vi "GUI_Cameras_v1.2.0_TEMP.vi"() -> ()   [LabVIEW 2013]
uses:
  <vilib>/vision/NI_Vision_Development_Module.lvlib
  <vilib>/Analysis/NI_AALBase.lvlib
  <vilib>/Analysis/baseanly.llb/Mean (DBL).vi
  <vilib>/Utility/miscctls.llb/LVRectTypeDef.ctl
panel:
  out "data array":dbl[](array[numeric])
  out "Guppy Y":dbl=985.6842015448223
  out "Guppy X":dbl=985.6842015448223
  out "M3 X":dbl=985.6842015448223
  out "M3 Y":dbl=985.6842015448223
  out "Image (Guppy)":T1(plugin-control)
  out "Image (OAP)":T1(plugin-control)
  in  "ROI":T2={"Global Rectangle"=[217, 150, 349, 397], "Contours"=[{"Contour Type"=0, "ROI Type"=3, "Points"=[217, 150, 349, 397]}, {"Contour Type"=0, "ROI Type"=3, "Points"=[382, 143, 522, 397]}, {"Contour Type"=0, "ROI Type"=3, "Points"=[555, 160, 687, 390]}]}
  out "Boolean":bool=TRUE
  out "time string":string="2:08 PM"
  in  "Search Decimal Separator":bool=TRUE
  out "Output value":dbl=2.5400000000000005 format="%.2f"
  in  "LCD/LED (LCD)":bool
  out "Segments status":T3(array[cluster])=[{TRUE, TRUE, FALSE, TRUE, TRUE, FALSE, TRUE}, {TRUE, FALSE, TRUE, TRUE, FALSE, TRUE, TRUE}, {FALSE, TRUE, TRUE, FALSE, FALSE, TRUE, TRUE}]
  out "error out 2":errorcluster
  in  "Threshold":dbl=3.0 format="%.2f"
  out "Zoom changed":bool
  out "Zoom old":cluster{"X":sgl, "Y":sgl}={"X"=1.2111253, "Y"=1.773196}
  out "MaxCounts":dbl(slide)=255.0 scale=0.0..256.0
  out "ratio(h)":bool=TRUE
  out "fixsize":bool
  out "Change Ratio":cluster{"X":sgl, "Y":sgl}={"X"=0.41283923, "Y"=0.28197673}
  out "old Panel Bounds":T4={"Left"=2, "Top"=-1034, "Right"=1328, "Bottom"=-402}
  in  "shotnumber":i32=32
  in  "gain":dbl
  in  "exposure":dbl=0.032 caption="Exposure"
  in  "save":bool
  in  "trigger":bool
  in  "triggerdelay":dbl
  out "error (h)":bool
  in  "Main Tap":T5(tab)=enum."Time"
  out "Image (IMAQ)":T1(plugin-control)
  out "output cluster":cluster{dbl[], dbl[]}[](graph)
  out "local Port":u16=65401
  out "Remote Host":string="192.168.10.115"
  out "port or service name":u16=65417
  in  "timeout ms (slow resp)":i32=500
  in  "reset":bool
  out "All Devices (h)":string[](array[string])=["StagingDiodeMonitor", "StagingFocusBeam1", "StagingFocusBeam2", "StagingGuppy", "StagingM1Far", "StagingM1Near", "StagingM3Far", "StagingOAP1Far", "StagingOAP1Near", "StagingOAP2Far", "StagingOAP2Near", "TS-InputNearField", "TS-Mode1"]
  out "centroidy":dbl=447.895874
  out "fast ID (h)":refnum<k16>
  out "slow ID (h)":refnum<k16>
  out "error out":errorcluster
  out "connections (hidden)":variant[](array[variant])=[variant(refnum<k16> refnum), variant(refnum<k16> refnum)]
  in  "time to wait (main loop)":i32=10
  in  "time to wait (TCP)":i32=10
  out "Data String":string="exposure,0.032000\r\ntrigger,off\r\nsave,off\r\ngain,0.000000\r\ntriggerdelay,0.000000\r\nlocalsavingpath,c:\\temp\r\ncentroidy,447.895874\r\ncentroidy,447.895874\r\n"
  in  "send":bool
  in  "localsavingpath":path=path "c:/temp"
  out "centroidy":dbl=447.895874
  out "Image (array)":u8[][](graph)
  out "Device Name (h)":string="StagingFocusBeam1"
  out "stop":bool
  out "error message":string
  out "image connection":bool=TRUE
  out "data connection ok":bool=TRUE
  # "Data"
  # "Image"
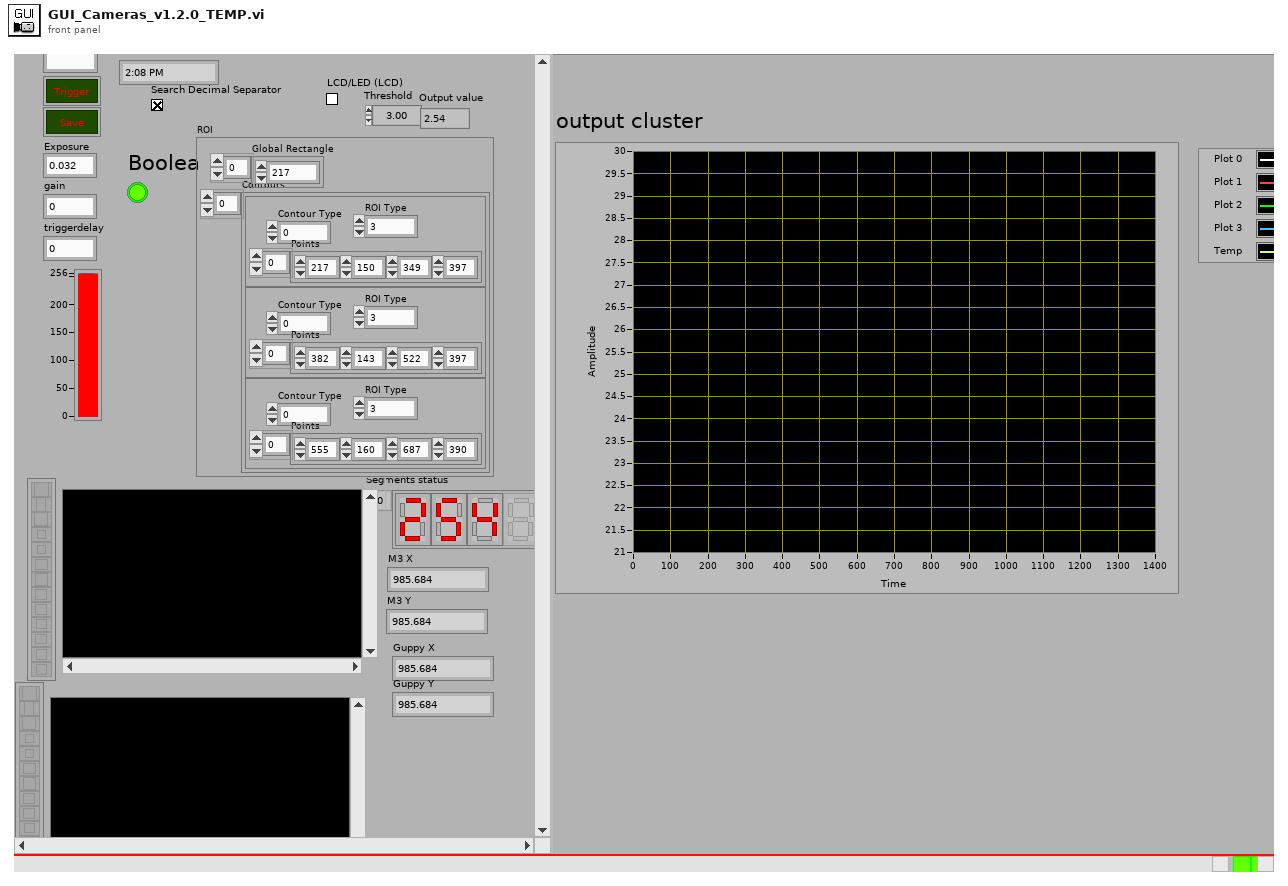
[diagram p1: front panel]
types:
  T1 = typedef "IMAQ Image.ctl" = refnum<image>
  T2 = cluster{"Global Rectangle":i32[], "Contours":cluster{"Contour Type":u32, "ROI Type":u32, "Points":i32[]}[]}
  T3 = cluster{bool, bool, bool, bool, bool, bool, bool}[]
  T4 = typedef "LVRectTypeDef.ctl" = cluster{"Left":i16, "Top":i16, "Right":i16, "Bottom":i16}
  T5 = enum32{"IMAQ", "Time", "Network", "Internal", "Array"}
  T6 = enum16{"Grayscale", "Binary", "Gradient", "Rainbow", "Temperature", "User Defined"}
  T7 = typedef "Image Type" = u32
  T8 = typedef "ROI Descriptor" = cluster{"Global Rectangle":i32[], "Contours":cluster{"ID":enum32{"External", "Internal"}, "Type":u32, "Coordinates":i32[]}[]}
  T9 = typedef "LVBoundsTypeDef.ctl" = cluster{"Width":u32, "Height":u32}
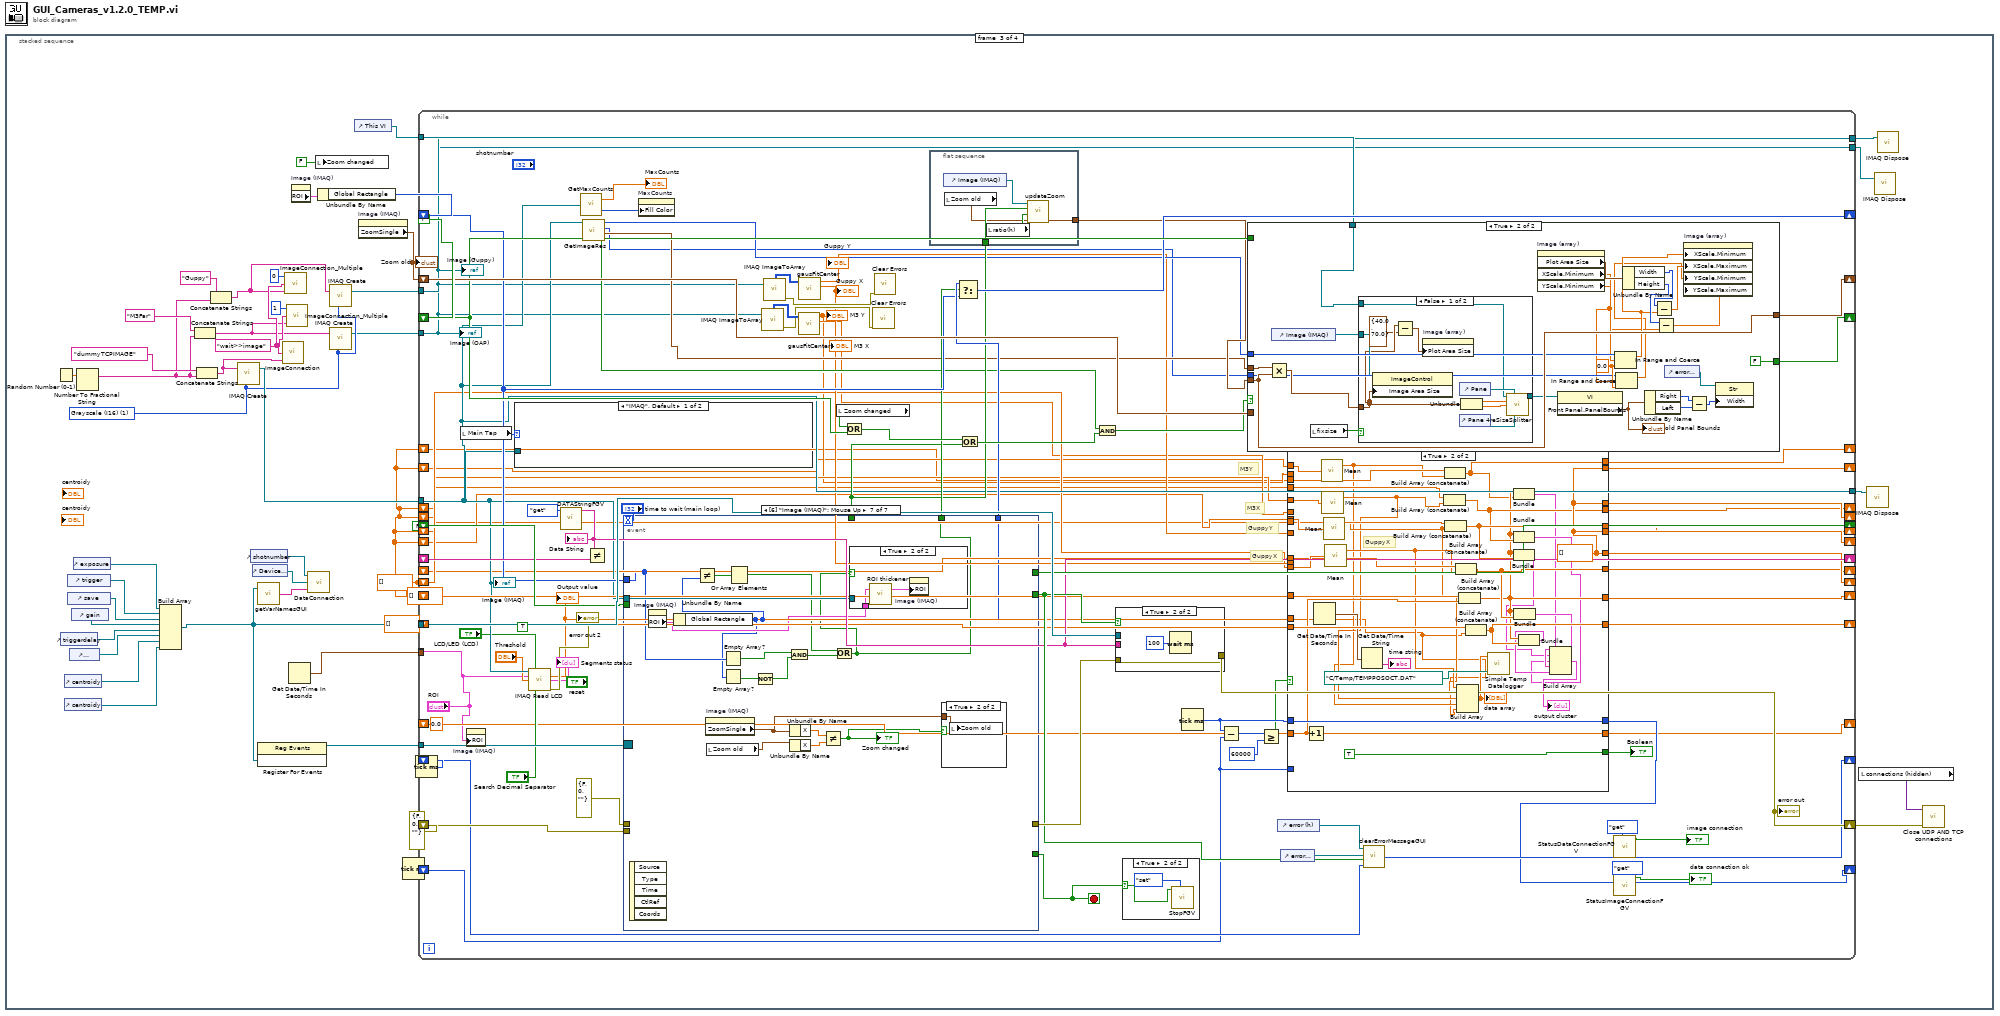
[diagram p0: block diagram]
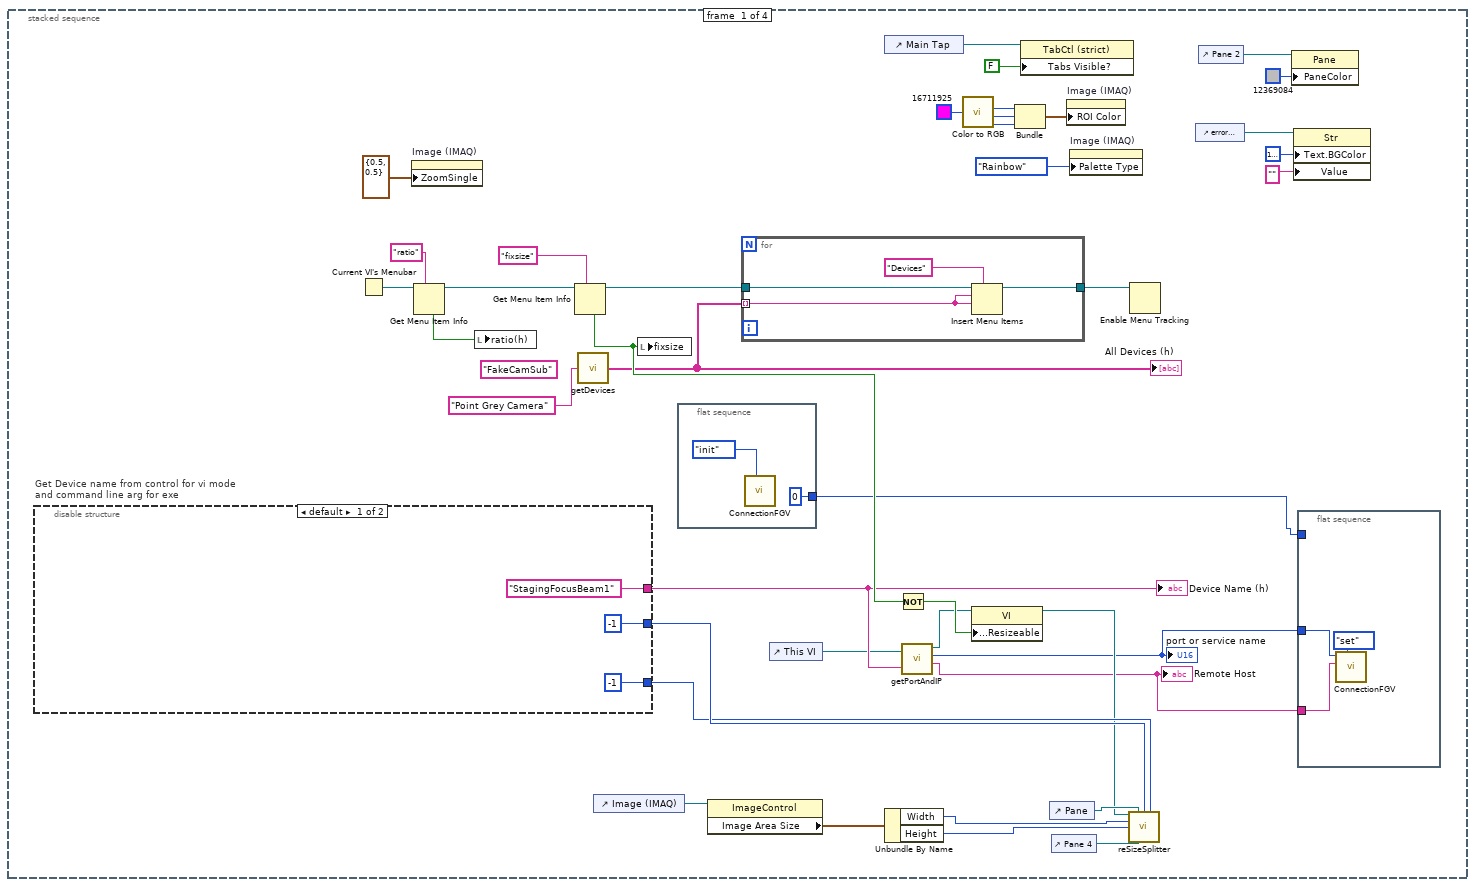
[diagram p2: hidden frame]
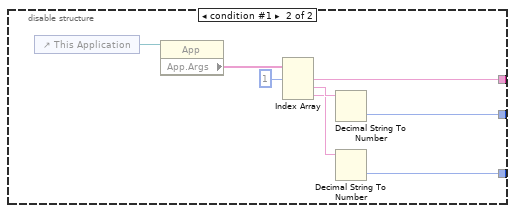
[diagram p3: hidden frame]
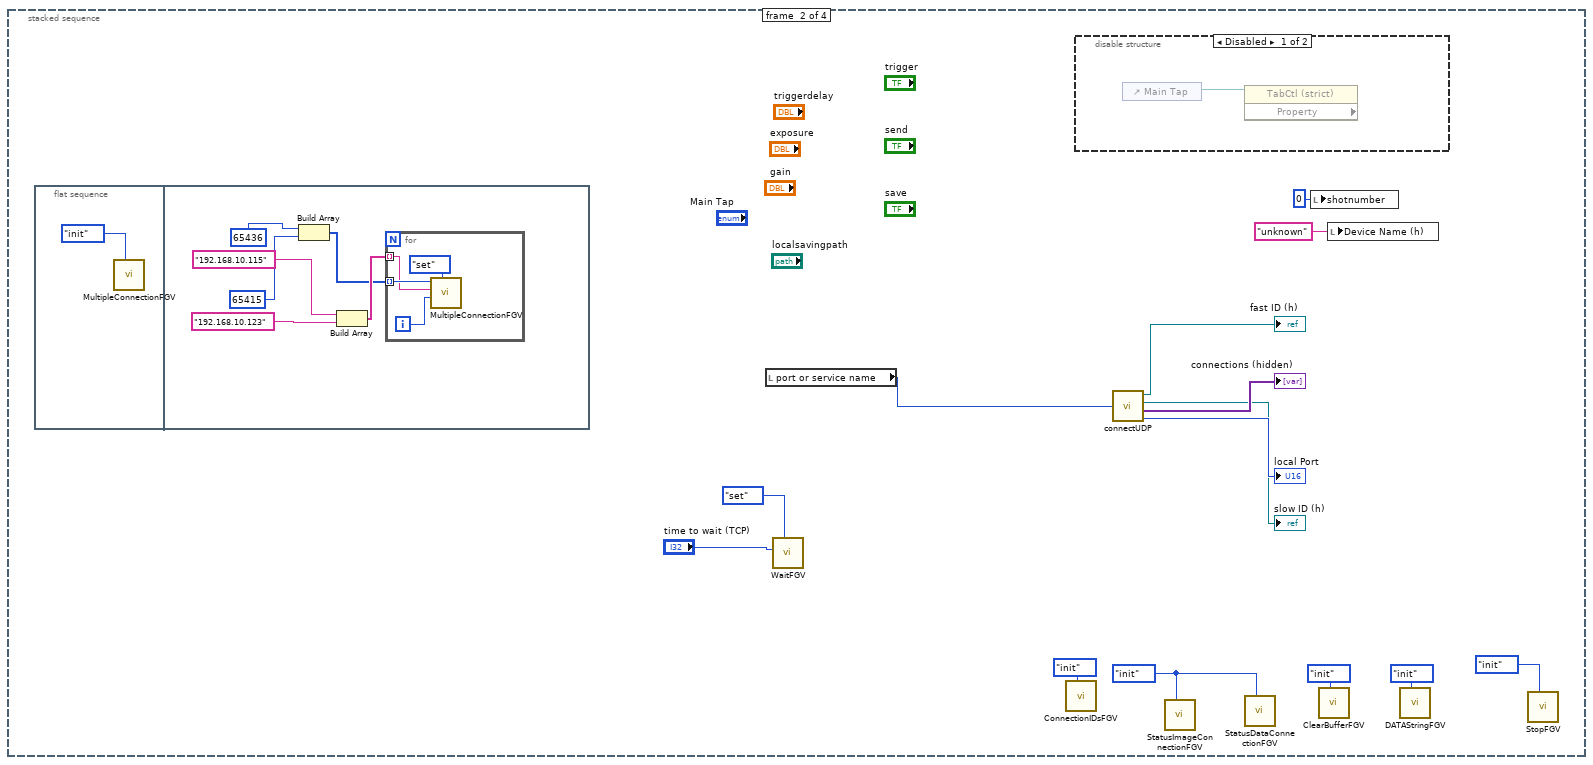
[diagram p4: hidden frame]
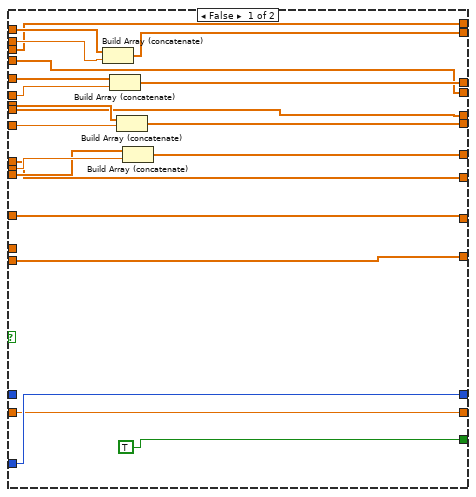
[diagram p6: hidden frame]
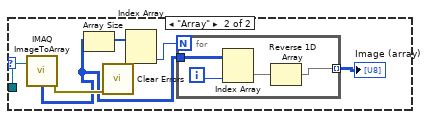
[diagram p8: hidden frame]
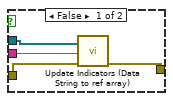
[diagram p11: hidden frame]
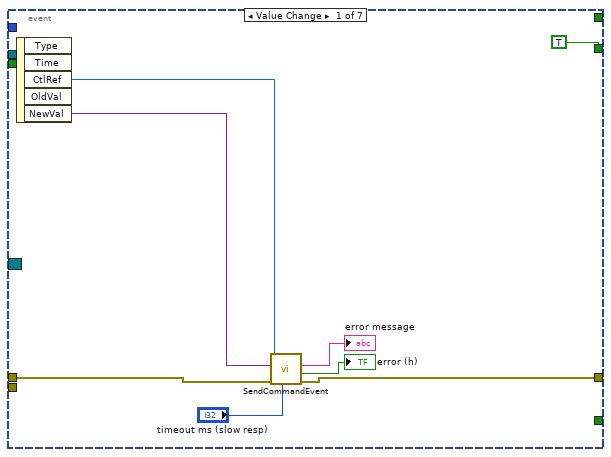
[diagram p12: hidden frame]
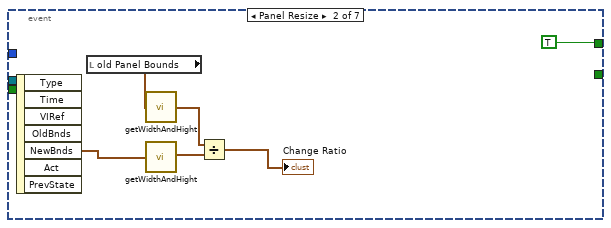
[diagram p13: hidden frame]
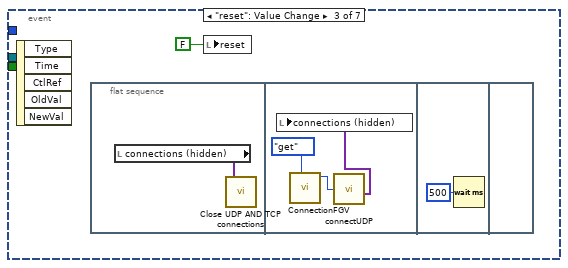
[diagram p14: hidden frame]
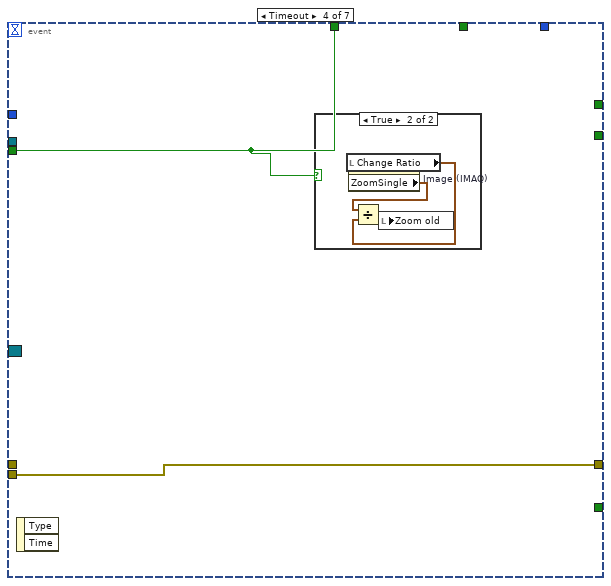
[diagram p15: hidden frame]
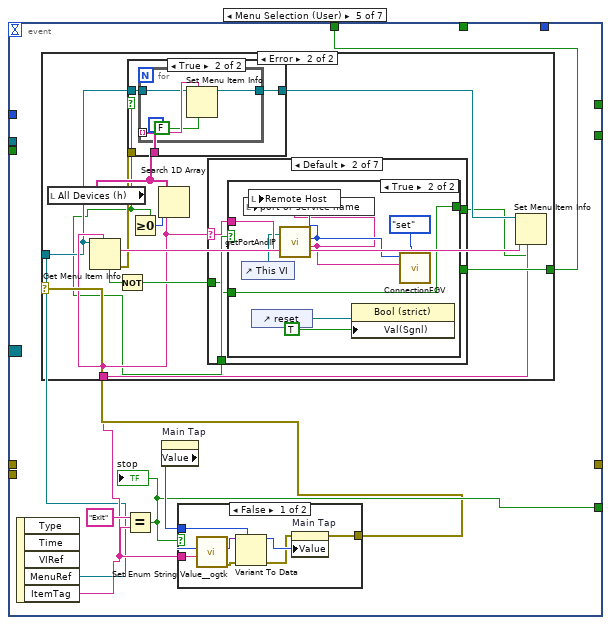
[diagram p17: hidden frame]
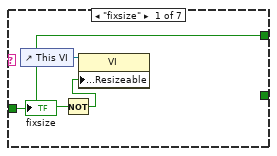
[diagram p20: hidden frame]
diagram:
  n1 = stacked-sequence {
    frame #0 {
      (unwired) "FakeCamSub" ("Device Class")
      n2 = disable-structure "Get Device name from control for vi mode\nand command line arg for exe" shown="default" {
        disable-tunnel: ["StagingFocusBeam1" ("Device Name for vi mode") w57] -> w14
        disable-tunnel: [i16 -1 ("left") w54] -> w27
        disable-tunnel: [i16 -1 ("left") w53] -> w26
        frame condition #0 (active) {
        }
        frame condition #1 {
          n3 = control-ref of="This Application"() -> (w60:refnum<vi>)
          n4 = property class="App"(reference=w60) -> ("App.Args"=w59:string[])  [unwired: 1 in, 2 out]
          n5 = Index Array(array=w59, index #1=1 ("index")) -> (element #1=w57:string, element #2=w56:string, element #3=w55:string)  [unwired: 2 in]
          n6 = Decimal String To Number(string=w56) -> (number=w54:i32)  [unwired: 2 in, 1 out]
          n7 = Decimal String To Number(string=w55) -> (number=w53:i32)  [unwired: 2 in, 1 out]
        }
      }
      "Device Name (h)" <- w14
      n8 = Current VI's Menubar() -> (w31:refnum<k9>)
      n9 = property on="Image (IMAQ)" class="ImageControl"("ZoomSingle"=cluster{"X":sgl, "Y":sgl} {"X"=0.5, "Y"=0.5} ("ZoomSingle:All Elements")) -> ()  [unwired: 2 in, 2 out]
      n10 = Get Menu Item Info(7:"ratio" ("item tag"), 11:w31) -> (3:w29:refnum<k9>, 4:w30:bool)  [unwired: 1 in, 5 out]
      n11 = local write "ratio(h)"(w30) -> ()
      n12 = Get Menu Item Info(7:"fixsize" ("item tag"), 11:w29) -> (3:w17:refnum<k9>, 4:w24:bool)  [unwired: 1 in, 5 out]
      n13 = call "getDevices.vi"("Device Class"="Point Grey Camera") -> ("All Devices"=w15:string[])
      "All Devices (h)" <- w15
      n14 = control-ref of="Image (IMAQ)"() -> (w38:refnum<vi>)
      n15 = local write "fixsize"(w24) -> ()
      n16 = flat-sequence {
        tunnel: [0] -> w1
        frame #0 {
          n17 = call "ConnectionFGV.vi"("command"=enum16{"get", "set", "init"}."init") -> ()  [unwired: 9 in, 2 out]
        }
      }
      n18 = property class="ImageControl"(reference=w38) -> ("Image Area Size"=w37:cluster{"Width":u32, "Height":u32})  [unwired: 1 in, 2 out]
      n19 = for {
        tunnel: w17 -> [w49]
        tunnel: [w48] -> w16
        tunnel: w15 -> [w46] mode=indexing
        n20 = Insert Menu Items(5:"Devices" ("menu tag"), 7:w46, 8:w46, 9:w49) -> (3:w48:refnum<k9>)  [unwired: 2 in, 2 out]
      }
      n21 = control-ref of="This VI"() -> (w13:refnum<vi>)
      n22 = control-ref of="Main Tap"() -> (w40:refnum<vi>)
      n23 = Unbundle By Name(w37) -> ("Width"=w36:u32, "Height"=w35:u32)
      n24 = Not(x=w24) -> (.not. x?=w25:bool)
      n25 = call "getPortAndIP.vi"("This Vi"=w13, "Device Name"=w14) -> ("reference out"=w12:refnum<vi>, "port or service name"=w4:u16, "Remote Host"=w3:string)  [unwired: 1 in]
      "port or service name" <- w4
      "Remote Host" <- w3
      n26 = call <vilib>:"Color to RGB.vi"("Color"=u32 16711925) -> ("R"=w9:u8, "G"=w8:u8, "B"=w7:u8)  [unwired: 1 out]
      n27 = property class="VI"(reference=w12, "Front Panel.Resizeable"=w25) -> (reference out=w5:refnum<vi>)  [unwired: 1 in, 1 out]
      n28 = Bundle("R"=w9, "G"=w8, "B"=w7) -> (w6:cluster{"R":u8, "G":u8, "B":u8})  [unwired: 1 in]
      n29 = property class="TabCtl (strict)"(reference=w40, "Tabs Visible?"=FALSE) -> ()  [unwired: 1 in, 2 out]
      n30 = control-ref of="Pane"() -> (w34:refnum<vi>)
      n31 = control-ref of="Pane 4"() -> (w23:refnum<vi>)
      n32 = property on="Image (IMAQ)" class="ImageControl"("ROI Color"=w6) -> ()  [unwired: 2 in, 2 out]
      n33 = property on="Image (IMAQ)" class="ImageControl"("Palette Type"=T6."Rainbow" ("Palette:Palette Type")) -> ()  [unwired: 2 in, 2 out]
      n34 = call "reSizeSplitter.vi"("this vi"=w5, "pane"=w34, "left"=w27, "top"=w26, "Width"=w36, "Height"=w35, "pane2"=w23) -> ()  [unwired: 8 in, 1 out]
      n35 = Enable Menu Tracking(4:w16) -> ()  [unwired: 2 in, 2 out]
      n36 = control-ref of="error message"() -> (w21:refnum<vi>)
      n37 = control-ref of="Pane 2"() -> (w19:refnum<vi>)
      n38 = property class="Pane"(reference=w19, "PaneColor"=u32 12369084) -> ()  [unwired: 1 in, 2 out]
      n39 = property class="Str"(reference=w21, "Text.BGColor"=u32 16777238, "Value"="") -> ()  [unwired: 1 in, 2 out]
      n40 = flat-sequence {
        tunnel: w4 -> [w42]
        tunnel: w3 -> [w41]
        tunnel: w1 -> [_]
        frame #0 {
          n41 = call "ConnectionFGV.vi"("command"=enum16{"get", "set", "init"}."set", "Remote Host in"=w41, "port or service name in"=w42) -> ()  [unwired: 7 in, 2 out]
        }
      }
    }
    frame #1 {
      w70 = enum16{"get", "set", "init"}."init" ("Command")
      n42 = flat-sequence {
        frame #0 {
          n43 = call "MultipleConnectionFGV.vi"("command"=enum16{"get", "set", "init"}."init") -> ()  [unwired: 9 in, 2 out]
        }
        frame #1 {
          n44 = Build Array(u16 65436 ("port or service name"), u16 65415 ("port or service name")) -> (w80:u16[])
          n45 = Build Array("192.168.10.115" ("Remote Host"), "192.168.10.123" ("Remote Host")) -> (w81:string[])
          n46 = for {
            tunnel: w80 -> [w84] mode=indexing
            tunnel: w81 -> [w83] mode=indexing
            i -> [w82]
            n47 = call "MultipleConnectionFGV.vi"("command"=enum16{"get", "set", "init"}."set", "Nr."=w82, "Remote Host in"=w83, "port or service name in"=w84) -> ()  [unwired: 6 in, 2 out]
          }
        }
      }
      n48 = local read "port or service name"() -> (w72:u16)
      n49 = call "WaitFGV.vi"("Command"=enum16{"get", "set", "init"}."set", "milliseconds to wait"="time to wait (TCP)") -> ()  [unwired: 9 in, 1 out]
      n50 = call "ConnectionIDsFGV.vi"("Command"=enum16{"add", "get", "init"}."init") -> ()  [unwired: 10 in, 1 out]
      n51 = disable-structure shown="Disabled" {
        frame Disabled {
          n52 = control-ref of="Main Tap"() -> (w86:refnum<vi>)
          n53 = property class="TabCtl (strict)" props=[](reference=w86) -> ()  [unwired: 1 in, 3 out]
        }
        frame Enabled {
        }
      }
      n54 = call "connectUDP.vi"("port or service name NOT USED"=w72) -> ("fast ID (h)"=→"fast ID (h)":refnum<k16>, "slow ID (h)"=→"slow ID (h)":refnum<k16>, "connections (hidden)"=→"connections (hidden)":variant[], "local Port"=→"local Port":u16)
      n55 = call "StatusImageConnectionFGV.vi"("Command"=w70) -> ()  [unwired: 10 in, 1 out]
      n56 = call "StatusDataConnectionFGV.vi"("Command"=w70) -> ()  [unwired: 10 in, 1 out]
      n57 = local write "shotnumber"(0 ("shotnumber")) -> ()
      n58 = call "ClearBufferFGV.vi"("Command"=enum16{"set", "get", "init"}."init") -> ()  [unwired: 10 in, 1 out]
      n59 = local write "Device Name (h)"("unknown" ("Device Name")) -> ()
      n60 = call "DATAStringFGV.vi"("Command"=enum16{"get", "set", "init"}."init") -> ()  [unwired: 9 in, 2 out]
      n61 = call "StopFGV.vi"("Command"=enum16{"set", "get", "init"}."init") -> ()  [unwired: 9 in, 2 out]
    }
    frame #2 {
      w87 = dbl[] []
      w99 = "wait>>image" ("Image Subscriber list")
      w98 = T7 1 items=["Grayscale (U8)", "Grayscale (I16)", "Grayscale (SGL)", "Complex (CSG)", "RGB (U32)", "HSL (U32)", "RGB (U64)", "Grayscale (U16)"] ("Image Type")
      n62 = Random Number (0-1)() -> (number: 0 to 1=w130:dbl)
      n63 = control-ref of="triggerdelay"() -> (w122:refnum<vi>)
      n64 = control-ref of="centroidy"() -> (w116:refnum<vi>)
      n65 = control-ref of="centroidy"() -> (w109:refnum<vi>)
      n66 = control-ref of="trigger"() -> (w126:refnum<vi>)
      n67 = control-ref of="save"() -> (w124:refnum<vi>)
      n68 = control-ref of="localsavingpath"() -> (w117:refnum<vi>)
      n69 = control-ref of="gain"() -> (w123:refnum<vi>)
      n70 = control-ref of="exposure"() -> (w125:refnum<vi>)
      n71 = Number To Fractional String(number=w130) -> (F-format string=w90:string)  [unwired: 3 in]
      n72 = Build Array(w125, w126, w124, w123, w122, w117, w116, w109) -> (w107:refnum<vi>[])
      n73 = Concatenate Strings("M3Far" ("Image Name"), w90) -> (w89:string)
      n74 = Concatenate Strings("dummyTCPIMAGE" ("Image Name"), w90) -> (w128:string)
      n75 = Concatenate Strings("Guppy" ("Image Name"), w90) -> (w92:string)
      n76 = call "IMAQ Create"("Image Name"=w128, "Image Type"=w98) -> ("New Image"=w132:T1)  [unwired: 3 in, 1 out]
      n77 = control-ref of="shotnumber"() -> (w111:refnum<vi>)
      n78 = control-ref of="Device Name (h)"() -> (w110:refnum<vi>)
      n79 = call "getVarNamesGUI.vi"("Array"=w107) -> ("String"=w106:string)  [unwired: 1 in]
      n80 = register-events(w107) -> (reference out=w108:refnum<event-registration>)  [unwired: 2 in, 1 out]
      n81 = call "ImageConnection.vi"("Image Name"=w128, "Image Subscriber list"=w99) -> ()  [unwired: 2 in]
      n82 = call "ImageConnection_Multiple.vi"("Image Name"=w92, "Image Subscriber list"=w99, "Nr."=0) -> ()  [unwired: 1 in]
      n83 = call "ImageConnection_Multiple.vi"("Image Name"=w89, "Image Subscriber list"=w99, "Nr."=1) -> ()  [unwired: 1 in]
      n84 = Get Date/Time In Seconds() -> (seconds since 1Jan1904=w105:timestamp)
      n85 = property on="Image (IMAQ)" class="ImageControl"() -> ("ROI"=w115:T2)  [unwired: 2 in, 2 out]
      n86 = call "DataConnection.vi"("Subscriber list"=w106, "Device Name (h)"=w110, "shotnumber"=w111) -> ()
      n87 = local write "Zoom changed"(FALSE ("Zoom changed")) -> ()
      n88 = Unbundle By Name(w115) -> ("Global Rectangle"=w114:i32[])
      n89 = call "IMAQ Create"("Image Name"=w92, "Image Type"=w98) -> ("New Image"=w97:T1)  [unwired: 3 in, 1 out]
      n90 = call "IMAQ Create"("Image Name"=w89, "Image Type"=w98) -> ("New Image"=w96:T1)  [unwired: 3 in, 1 out]
      n91 = control-ref of="This VI"() -> (w113:refnum<vi>)
      n92 = property on="Image (IMAQ)" class="ImageControl"() -> ("ZoomSingle"=w121:cluster{"X":sgl, "Y":sgl})  [unwired: 2 in, 2 out]
      "Zoom old" <- w121
      n93 = Tick Count (ms)() -> (millisecond timer value=w103:u32)
      n94 = Tick Count (ms)() -> (millisecond timer value=w118:u32)
      n95 = while {
        shift-right: [w220] -> w131
        shift-left: errorcluster {"status"=FALSE, "code"=0, "source"=""} ("error out") -> [w222]
        tunnel: w132 -> [w164]
        tunnel: [w164] -> w133
        tunnel: w107 -> [w224]
        shift-right: [w219] -> _
        shift-left: w121 -> [w218]
        shift-right: [w216] -> _
        shift-left: FALSE -> [w217]
        shift-right: [w215] -> _
        shift-left: TRUE -> [w214]
        shift-right: [w210] -> _
        shift-left: w118 -> [w209]
        shift-right: [w184] -> _
        shift-left: _ -> [w207]
        shift-right: [w203] -> _
        shift-left: w114 -> [w202]
        tunnel: w113 -> [w200]
        tunnel: w108 -> [w182]
        tunnel: ["ROI"] -> _
        tunnel: w105 -> [_]
        shift-right: [w176] -> _
        shift-left: dbl[] [] -> [w165]
        shift-right: [w178] -> _
        shift-left: dbl[] [] ("Array") -> [w177]
        shift-right: [w169] -> _
        shift-left: w103 -> [w171]
        shift-right: [w167] -> _
        shift-left: 0.0 -> [w166]
        tunnel: w97 -> [w160]
        tunnel: w96 -> [w159]
        tunnel: [w159] -> w94
        tunnel: [w160] -> w95
        shift-right: [w153] -> _
        shift-left: w87 -> [w152]
        shift-right: [w151] -> _
        shift-left: w87 -> [w150]
        shift-right: [w148] -> _
        shift-left: w87 -> [w147]
        shift-right: [w146] -> _
        shift-left: w87 -> [w145]
        shift-right: [w143] -> _
        shift-left: w87 -> [w142]
        shift-right: [w141] -> _
        shift-left: w87 -> [w140]
        shift-right: [w136] -> _
        shift-left: w87 -> [w135]
        shift-right: [w138] -> _
        shift-left: w87 -> [w137]
        stop <- w185 stop-if-true
        (unwired) TRUE ("LCD / LED (LCD)")
        # "M3Y"
        # "M3X"
        # "GuppyY"
        # "GuppyX"
        n96 = local read "Main Tap"() -> (w205:T5)
        n97 = property on="Image (IMAQ)" class="ImageControl"("ROI"="ROI") -> ()  [unwired: 2 in, 2 out]
        n98 = case shown="\"IMAQ\", Default" w205 {
          tunnel: w164 -> [_ w295]
          frame "IMAQ", Default {
          }
          frame "Array" {
            n99 = call "IMAQ ImageToArray"("Image"=w295) -> ("error out"=w294:errorcluster, "Image Pixels (U8)"=w291:u8[][])  [unwired: 3 in, 3 out]
            n100 = Array Size(array=w291) -> (size(s)=w293:i32[])
            n101 = call <vilib>:"Clear Errors.vi"("error in (no error)"=w294) -> ()  [unwired: 6 in, 1 out]
            n102 = Index Array(array=w293) -> (element #2=w290:i32)  [unwired: 2 in, 1 out]
            n103 = for {
              N: w290 -> [_]
              tunnel: w291 -> [w299]
              tunnel: [w297] -> w292 mode=indexing
              i -> [w296]
              n104 = Index Array(array=w299, index (col)=w296) -> (element=w298:u8[])  [unwired: 1 in]
              n105 = Reverse 1D Array(array=w298) -> (reversed array=w297:u8[])
            }
            "Image (array)" <- w292
          }
        }
        n106 = call "IMAQ Read LCD"("Image"=w164, "LCD/LED (LCD)"="LCD/LED (LCD)", "ROI Descriptor"="ROI", "Threshold"="Threshold", "Search Decimal Separator"="Search Decimal Separator") -> ("Output value"=w175:dbl, "Segments status"=→"Segments status":T3, "error out"=→"error out 2":errorcluster)  [unwired: 7 in, 1 out]
        "Output value" <- w175
        n107 = call "DATAStringFGV.vi"("Command"=enum16{"get", "set", "init"}."get") -> ("Data String out"=w184:string)  [unwired: 9 in, 1 out]
        "Data String" <- w184
        n108 = call "GetMaxCounts.vi"("New Image"=w164) -> ("Maximal Value"=→"MaxCounts":sgl, "Color"=w196:u32)
        n109 = call "GetImageRes.vi"("Image"=w164) -> ("valid Image"=w193:bool, "Image Area:Size:All Elements"=w194:cluster{"Width":u32, "Height":u32}, "Y Resolution"=w191:i32, "X Resolution"=w192:i32)  [unwired: 6 in, 1 out]
        n110 = Not Equal?(x=w184, y=w207) -> ()  [unwired: 1 out]
        n111 = event shown="[6] \"Image (IMAQ)\": Mouse Up" {
          selector: w182 -> [_ _ _ _ _ _ _]
          dyn-events: _ -> [_ _ _ _ _ _ _]
          timeout: "time to wait (main loop)" -> [_ _ _ _ _ _ _]
          tunnel: [w349 _ _ w365 _ _ _] -> w221
          tunnel: errorcluster {"status"=FALSE, "code"=0, "source"=""} ("error out") -> [w351 _ _ _ _ _ _]
          tunnel: w222 -> [_ _ _ w365 _ _ _]
          tunnel: [TRUE _ _ _ _ _ _] -> w206
          tunnel: [_ _ _ _ w373 _ _] -> w185
          tunnel: [_ _ _ w364 w370 _ _] -> w199
          tunnel: w217 -> [_ _ _ w364 _ _ _]
          tunnel: [_ TRUE _ _ _ _ _] -> w216
          tunnel: [_ _ _ _ _ _ w451] -> w204
          tunnel: w202 -> [_ _ _ _ _ _ w452]
          tunnel: [_ _ _ _ _ _ w445] -> w201
          tunnel: w164 -> [_ _ _ _ _ _ w454]
          event Value Change {
            n112 = event-data() -> ("CtlRef"=w346:refnum<vi>, "NewVal"=w345:variant)  [unwired: 1 in, 3 out]
            n113 = call "SendCommandEvent.vi"("timeout ms (slow resp)"="timeout ms (slow resp)", "error out 2"=w351, "NewVal"=w345, "CtlRef"=w346) -> ("error out"=w349:errorcluster, "error (h)"=→"error (h)":bool, "error message"=→"error message":string)  [unwired: 4 in, 1 out]
          }
          event Panel Resize {
            n114 = event-data() -> ("NewBnds"=w357:T4)  [unwired: 1 in, 6 out]
            n115 = local read "old Panel Bounds"() -> (w355:T4)
            n116 = call "getWidthAndHight.vi"("OldBnds"=w355) -> ("output cluster"=w354:cluster{"X":sgl, "Y":sgl})
            n117 = call "getWidthAndHight.vi"("OldBnds"=w357) -> ("output cluster"=w353:cluster{"X":sgl, "Y":sgl})
            n118 = Divide(x=w354, y=w353) -> (x/y=→"Change Ratio":cluster{"X":sgl, "Y":sgl})
          }
          event "reset": Value Change {
            n119 = event-data() -> ()  [unwired: 1 in, 5 out]
            n120 = flat-sequence {
              frame #0 {
                n121 = local read "connections (hidden)"() -> (w359:variant[])
                n122 = call "Close UDP AND TCP connections.vi"("appended array"=w359) -> ()  [unwired: 7 in]
              }
              frame #1 {
                n123 = call "ConnectionFGV.vi"("command"=enum16{"get", "set", "init"}."get") -> ("port or service name out"=w361:u16)  [unwired: 9 in, 1 out]
                n124 = call "connectUDP.vi"("port or service name NOT USED"=w361) -> ("connections (hidden)"=w360:variant[])  [unwired: 3 out]
                n125 = local write "connections (hidden)"(w360) -> ()
              }
              frame #2 {
                n126 = Wait (ms)(milliseconds to wait=u32 500) -> ()  [unwired: 1 out]
              }
              frame #3 {
              }
            }
            n127 = local write "reset"(FALSE ("reset")) -> ()
          }
          event Timeout {
            n128 = event-data() -> ()  [unwired: 1 in, 2 out]
            n129 = case shown="True" w364 {
              frame False {
              }
              frame True {
                n130 = local read "Change Ratio"() -> (w367:cluster{"X":sgl, "Y":sgl})
                n131 = property on="Image (IMAQ)" class="ImageControl"() -> ("ZoomSingle"=w368:cluster{"X":sgl, "Y":sgl})  [unwired: 2 in, 2 out]
                n132 = Divide(x=w368, y=w367) -> (x/y=w366:cluster{"X":sgl, "Y":sgl})
                n133 = local write "Zoom old"(w366) -> ()
              }
            }
          }
          event Menu Selection (User) {
            n134 = event-data() -> ("MenuRef"=w369:refnum<k9>, "ItemTag"=w371:string)  [unwired: 1 in, 3 out]
            n135 = Equal?(x="Exit", y=w371) -> (x = y?=w373:bool)
            "stop" <- w373
            n136 = property on="Main Tap" class="TabCtl (strict)"() -> ("Value"=w375:T5)  [unwired: 2 in, 2 out]
            n137 = case shown="False" w373 {
              tunnel: w375 -> [w434 _]
              tunnel: w371 -> [w433 _]
              tunnel: [w430 errorcluster {"status"=FALSE, "code"=0, "source"=""} ("error out")] -> w372
              frame False {
                n138 = call <userlib>:"Set Enum String Value__ogtk.vi"("String Value"=w433, "Default Enum Value"=w434) -> ("error out"=w432:errorcluster, "Enum"=w436:variant)  [unwired: 8 in]
                n139 = Variant To Data(error in=w432, type=w434, Variant=w436) -> (data=w435:T5, error out=w431:errorcluster)
                n140 = property on="Main Tap" class="TabCtl (strict)"(error in=w431, "Value"=w435) -> (error out=w430:errorcluster)  [unwired: 1 in, 1 out]
              }
              frame True {
              }
            }
            n141 = case shown="Error" w372 {
              tunnel: w369 -> [_ w379]
              tunnel: w371 -> [_ w383]
              tunnel: [_ w384] -> w370
              frame No Error {
              }
              frame Error {
                n142 = local read "All Devices (h)"() -> (w381:string[])
                n143 = Get Menu Item Info(7:w383, 11:w379) -> (0:w380:errorcluster, 2:w386:string, 4:w387:bool)  [unwired: 1 in, 4 out]
                n144 = Not(x=w387) -> (.not. x?=w385:bool)
                n145 = Search 1D Array(1D array=w381, element=w383) -> (index of element=w382:i32)  [unwired: 1 in]
                n146 = Greater Or Equal To 0?(x=w382) -> (x >= 0?=w378:bool)
                n147 = case shown="True" w378 {
                  tunnel: w381 -> [_ w391]
                  tunnel: w380 -> [_ _]
                  tunnel: w379 -> [w388 w390]
                  tunnel: [w388 w389] -> w377
                  frame False {
                  }
                  frame True {
                    n148 = for {
                      tunnel: w391 -> [w395] mode=indexing
                      tunnel: w390 -> [w393]
                      tunnel: [w392] -> w389
                      n149 = Set Menu Item Info(6:FALSE ("checked"), 7:w395, 11:w393) -> (3:w392:refnum<k9>)  [unwired: 4 in, 1 out]
                    }
                  }
                }
                n150 = case shown="Default" w383 {
                  selector: w383 -> [_ w401 _ _ w422 _ _]
                  tunnel: w385 -> [w396 w399 w412 _ _ _ w427]
                  tunnel: [_ _ TRUE _ _ _ _] -> w384
                  tunnel: w378 -> [_ w402 _ _ _ _ _]
                  tunnel: [w396 w400 w412 _ _ _ w427] -> w376
                  frame "fixsize" {
                    n151 = control-ref of="This VI"() -> (w398:refnum<vi>)
                    n152 = Not(x=w396) -> (.not. x?=w397:bool)
                    n153 = property class="VI"(reference=w398, "Front Panel.Resizeable"=w397) -> ()  [unwired: 1 in, 2 out]
                    "fixsize" <- w396
                  }
                  frame Default {
                    n154 = case shown="True" w402 {
                      tunnel: w401 -> [_ w410]
                      tunnel: [_ w406] -> w400
                      tunnel: w399 -> [_ w406]
                      frame False {
                      }
                      frame True {
                        n155 = control-ref of="This VI"() -> (w409:refnum<vi>)
                        n156 = control-ref of="reset"() -> (w408:refnum<vi>)
                        n157 = call "getPortAndIP.vi"("This Vi"=w409, "Device Name"=w410) -> ("port or service name"=w404:u16, "Remote Host"=w403:string)  [unwired: 1 in, 1 out]
                        n158 = local write "port or service name"(w404) -> ()
                        n159 = local write "Remote Host"(w403) -> ()
                        n160 = property class="Bool (strict)"(reference=w408, "Val(Sgnl)"=TRUE ("Value (Signaling)")) -> ()  [unwired: 1 in, 2 out]
                        n161 = call "ConnectionFGV.vi"("command"=enum16{"get", "set", "init"}."set", "Remote Host in"=w403, "port or service name in"=w404) -> ()  [unwired: 7 in, 2 out]
                      }
                    }
                  }
                  frame "ratio" {
                    n162 = property on="Image (IMAQ)" class="ImageControl"() -> ("ZoomSingle"=w411:cluster{"X":sgl, "Y":sgl})  [unwired: 2 in, 2 out]
                    n163 = local write "Zoom old"(w411) -> ()
                    "ratio(h)" <- w412
                  }
                  frame "Local Saving Path" {
                    n164 = control-ref of="localsavingpath"() -> (w414:refnum<vi>)
                    n165 = property class="Path"(reference=w414) -> (reference out=w417:refnum<vi>, "Value"=w418:path)  [unwired: 1 in, 1 out]
                    n166 = call "changePath.vi"("Local Saving in (h)"=w418) -> ("change (h)"=w416:bool, "Local Saving out (h)"=w415:path)  [unwired: 9 in]
                    n167 = case shown="True" w416 {
                      tunnel: w417 -> [_ w420]
                      tunnel: w415 -> [_ w419]
                      frame False {
                      }
                      frame True {
                        n168 = property class="Path"(reference=w420, "Val(Sgnl)"=w419) -> ()  [unwired: 1 in, 2 out]
                      }
                    }
                  }
                  frame "Binary", "Gradient", "Grayscale", "Rainbow", "Temperature" {
                    n169 = Scan From String(input string=w422, default 1=T6."Grayscale" ("Palette:Palette Type")) -> (output 1=w421:T6)  [unwired: 3 in, 3 out]
                    n170 = property on="Image (IMAQ)" class="ImageControl"("Palette Type"=w421) -> ()  [unwired: 2 in, 2 out]
                  }
                  frame "reset" {
                    n171 = control-ref of="reset"() -> (w425:refnum<vi>)
                    n172 = property class="Bool (strict)"(reference=w425, "Val(Sgnl)"=TRUE ("Value (Signaling)")) -> ()  [unwired: 1 in, 2 out]
                  }
                  frame "clear" {
                    n173 = control-ref of="reset"() -> (w429:refnum<vi>)
                    n174 = call "ClearBufferFGV.vi"("Command"=enum16{"set", "get", "init"}."set", "clear buffer"=w427) -> ()  [unwired: 9 in, 1 out]
                    n175 = property class="Bool (strict)"(reference=w429, "Val(Sgnl)"=TRUE ("Value (Signaling)")) -> ()  [unwired: 1 in, 2 out]
                  }
                }
                n176 = Set Menu Item Info(6:w376, 7:w383, 10:w386, 11:w377) -> ()  [unwired: 3 in, 2 out]
              }
            }
          }
          event "time to wait (TCP)": Value Change {
            n177 = event-data() -> ("NewVal"=w439:i32)  [unwired: 1 in, 4 out]
            n178 = call "WaitFGV.vi"("Command"=enum16{"get", "set", "init"}."set", "milliseconds to wait"=w439) -> ()  [unwired: 9 in, 1 out]
          }
          event "Image (IMAQ)": Mouse Up {
            n179 = event-data() -> ()  [unwired: 1 in, 5 out]
            n180 = property on="Image (IMAQ)" class="ImageControl"() -> ("ROI"=w453:T2)  [unwired: 2 in, 2 out]
            n181 = Unbundle By Name(w453) -> ("Global Rectangle"=w451:i32[])
            n182 = Not Equal?(x=w452, y=w451) -> (x != y?=w455:bool[])
            n183 = property on="Image (IMAQ)" class="ImageControl"() -> ("ZoomSingle"=w440:cluster{"X":sgl, "Y":sgl})  [unwired: 2 in, 2 out]
            n184 = local read "Zoom old"() -> (w442:cluster{"X":sgl, "Y":sgl})
            n185 = Empty Array?(array=w452) -> (empty?=w448:bool)
            n186 = Empty Array?(array=w451) -> (empty?=w450:bool)
            n187 = Or Array Elements(Boolean array=w455) -> (logical OR=w446:bool)
            n188 = Not(x=w450) -> (.not. x?=w449:bool)
            n189 = And(x=w448, y=w449) -> (x .and. y?=w447:bool)
            n190 = Unbundle By Name(w440) -> ("X"=w443:sgl)
            n191 = Unbundle By Name(w442) -> ("X"=w444:sgl)
            n192 = Not Equal?(x=w443, y=w444) -> (x != y?=w441:bool)
            "Zoom changed" <- w441
            n193 = Or(x=w446, y=w447) -> (x .or. y?=w445:bool)
            n194 = case shown="True" w445 {
              tunnel: w454 -> [_ _]
              tunnel: w453 -> [_ w458]
              frame False {
              }
              frame True {
                n195 = call "ROI thickener.vi"("ROI Descriptor in"=w458) -> ("ROI Descriptor out"=w457:T8)  [unwired: 1 in, 1 out]
                n196 = property on="Image (IMAQ)" class="ImageControl"("ROI"=w457) -> ()  [unwired: 2 in, 2 out]
              }
            }
            n197 = case shown="True" w441 {
              tunnel: w440 -> [_ w456]
              frame False {
              }
              frame True {
                n198 = local write "Zoom old"(w456) -> ()
              }
            }
          }
        }
        n199 = property on="MaxCounts" class="Slide (strict)"("Fill Color"=w196) -> ()  [unwired: 2 in, 2 out]
        n200 = call "IMAQ ImageToArray"("Image"=w159) -> ("error out"=w155:errorcluster, "Image Pixels (U8)"=w158:u8[][])  [unwired: 3 in, 3 out]
        n201 = call "IMAQ ImageToArray"("Image"=w160) -> ("error out"=w156:errorcluster, "Image Pixels (U8)"=w157:u8[][])  [unwired: 3 in, 3 out]
        n202 = call "gausFitCenter.vi"("Image Pixels (I16)"=w158) -> ("center 2"=w144:dbl, "center"=w139:dbl)  [unwired: 9 in]
        "M3 Y" <- w139
        "M3 X" <- w144
        n203 = call "gausFitCenter.vi"("Image Pixels (I16)"=w157) -> ("center 2"=w154:dbl, "center"=w149:dbl)  [unwired: 9 in]
        "Guppy X" <- w154
        "Guppy Y" <- w149
        n204 = local read "Zoom changed"() -> (w195:bool)
        n205 = Or(x=w195, y=w214) -> (x .or. y?=w213:bool)
        n206 = call <vilib>:"Clear Errors.vi"("error in (no error)"=w155) -> ()  [unwired: 6 in, 1 out]
        n207 = call <vilib>:"Clear Errors.vi"("error in (no error)"=w156) -> ()  [unwired: 6 in, 1 out]
        n208 = flat-sequence {
          tunnel: w199 -> [w288]
          tunnel: [w285] -> w198
          frame #0 {
            n209 = control-ref of="Image (IMAQ)"() -> (w289:refnum<vi>)
            n210 = local read "Zoom old"() -> (w286:cluster{"X":sgl, "Y":sgl})
            n211 = local read "ratio(h)"() -> (w287:bool)
            n212 = call "updateZoom.vi"("Zoom old"=w286, "ratio(h)"=w287, "update Zoom"=w288, "imageRef"=w289) -> ("Zoom out"=w285:cluster{"X":sgl, "Y":sgl})  [unwired: 7 in]
          }
        }
        n213 = Select(t=w204, s=w201, f=w202) -> (s? t:f=w203:i32[])
        n214 = Or(x=w213, y=w199) -> (x .or. y?=w211:bool)
        n215 = And(x=w193, y=w211) -> (x .and. y?=w212:bool)
        n216 = case shown="True" w206 {
          tunnel: w224 -> [w341 _]
          tunnel: w221 -> [w338 w343]
          tunnel: [w340 w343] -> w220
          tunnel: w184 -> [w339 _]
          frame False {
            n217 = call "Update Indicators (Data String to ref array).vi"("Array"=w341, "Data String"=w339, "error in (no error)"=w338) -> ("error out"=w340:errorcluster)  [unwired: 11 in, 1 out]
          }
          frame True {
            n218 = Wait (ms)(milliseconds to wait=u32 100) -> ()  [unwired: 1 out]
          }
        }
        "error out" <- w220
        n219 = case shown="True" w185 {
          selector: w185 -> [_ w283]
          frame False {
          }
          frame True {
            n220 = call "StopFGV.vi"("Command"=enum16{"set", "get", "init"}."set", "Stop"=w283) -> ()  [unwired: 8 in, 2 out]
          }
        }
        n221 = Tick Count (ms)() -> (millisecond timer value=w170:u32)
        n222 = Subtract(x=w170, y=w171) -> (x-y=w174:u32)
        n223 = case shown="True" w212 {
          tunnel: w198 -> [_ w325]
          tunnel: [w301 w325] -> w219
          tunnel: w218 -> [w301 _]
          tunnel: w194 -> [_ w326]
          tunnel: w214 -> [w300 _]
          tunnel: [w300 FALSE] -> w215
          tunnel: w192 -> [_ w310]
          tunnel: w191 -> [_ w306]
          tunnel: w200 -> [_ w303]
          frame False {
          }
          frame True {
            w307 = 0.0 ("lower limit")
            n224 = Multiply(x=w326, y=w325) -> (x*y=w324:cluster{sgl, sgl})
            n225 = control-ref of="Image (IMAQ)"() -> (w315:refnum<vi>)
            n226 = local read "fixsize"() -> (w316:bool)
            n227 = case shown="False" w316 {
              tunnel: w324 -> [w329 _]
              tunnel: w303 -> [w333 w337]
              tunnel: [w332 w337] -> w322
              tunnel: w315 -> [w331 _]
              frame False {
                n228 = property class="ImageControl"(reference=w331, "Image Area Size"=w329) -> ()  [unwired: 1 in, 2 out]
                n229 = Subtract(x=w329, y=cluster{sgl, sgl} {40.0, 70.0}) -> (x-y=w328:cluster{sgl, sgl})
                n230 = property on="Image (array)" class="IntGraph (strict)"("Plot Area Size"=w328) -> ()  [unwired: 2 in, 2 out]
                n231 = control-ref of="Pane"() -> (w334:refnum<vi>)
                n232 = control-ref of="Pane 4"() -> (w330:refnum<vi>)
                n233 = Unbundle(w329) -> (w335:sgl, w336:sgl)
                n234 = call "reSizeSplitter.vi"("this vi"=w333, "pane"=w334, "Width"=w335, "Height"=w336, "pane2"=w330) -> ("reference out"=w332:refnum<vi>)  [unwired: 10 in]
              }
              frame True {
              }
            }
            n235 = property on="Image (array)" class="IntGraph (strict)"() -> ("Plot Area Size"=w314:T9, "XScale.Minimum"=w308:dbl, "YScale.Minimum"=w305:dbl)  [unwired: 2 in, 2 out]
            n236 = property class="VI"(reference=w322) -> ("Front Panel.PanelBounds"=w321:T4)  [unwired: 1 in, 2 out]
            "old Panel Bounds" <- w321
            n237 = In Range and Coerce(upper limit=w310, x=w308, lower limit=w307) -> (coerced(x)=w309:dbl)  [unwired: 1 out]
            n238 = In Range and Coerce(upper limit=w306, x=w305, lower limit=w307) -> (coerced(x)=w304:dbl)  [unwired: 1 out]
            n239 = Unbundle By Name(w314) -> ("Width"=w313:u32, "Height"=w311:u32)
            n240 = Unbundle By Name(w321) -> ("Right"=w320:i16, "Left"=w319:i16)
            n241 = Subtract(x=w313, y=w309) -> (x-y=w312:dbl)
            n242 = Subtract(x=w311, y=w305) -> (x-y=w302:dbl)
            n243 = control-ref of="error message"() -> (w323:refnum<vi>)
            n244 = property on="Image (array)" class="IntGraph (strict)"("XScale.Minimum"=w309, "XScale.Maximum"=w312, "YScale.Minimum"=w304, "YScale.Maximum"=w302) -> ()  [unwired: 2 in, 2 out]
            n245 = Subtract(x=w320, y=w319) -> (x-y=w318:i16)
            n246 = property class="Str"(reference=w323, "Width"=w318) -> ()  [unwired: 1 in, 2 out]
          }
        }
        n247 = Greater Or Equal?(x=w174, y=u32 60000) -> (x >= y?=w168:bool)
        n248 = control-ref of="error (h)"() -> (w190:refnum<vi>)
        n249 = control-ref of="error message"() -> (w208:refnum<vi>)
        n250 = case shown="True" w168 {
          tunnel: [w244 w282] -> w178
          tunnel: w177 -> [w244 w281]
          tunnel: [w243 w262] -> w176
          tunnel: w175 -> [_ w247]
          tunnel: [TRUE TRUE] -> w172
          tunnel: w171 -> [w245 _]
          tunnel: w170 -> [_ w279]
          tunnel: [w245 w279] -> w169
          tunnel: [w242 w278] -> w167
          tunnel: w166 -> [w242 w277]
          tunnel: w165 -> [w243 w276]
          tunnel: w154 -> [w241 _]
          tunnel: [w240 w265] -> w153
          tunnel: w152 -> [w239 w275]
          tunnel: [w238 w273] -> w151
          tunnel: w150 -> [w238 w274]
          tunnel: w149 -> [w237 _]
          tunnel: [w236 w265] -> w148
          tunnel: w147 -> [w235 w271]
          tunnel: [w234 w264] -> w146
          tunnel: w145 -> [w234 w270]
          tunnel: w144 -> [w233 _]
          tunnel: [w232 w265] -> w143
          tunnel: w142 -> [w231 w269]
          tunnel: [w227 w263] -> w141
          tunnel: w140 -> [w227 w268]
          tunnel: w139 -> [w230 _]
          tunnel: [w229 w265] -> w138
          tunnel: w137 -> [w228 w267]
          tunnel: [w226 w261] -> w136
          tunnel: w135 -> [w226 w266]
          frame False {
            n251 = Build Array (concatenate)(w228, w230) -> (w229:dbl[])
            n252 = Build Array (concatenate)(w231, w233) -> (w232:dbl[])
            n253 = Build Array (concatenate)(w235, w237) -> (w236:dbl[])
            n254 = Build Array (concatenate)(w239, w241) -> (w240:dbl[])
          }
          frame True {
            w265 = dbl[] []
            # "GuppyX"
            n255 = Increment(x=w277) -> (x+1=w278:dbl)
            n256 = Get Date/Time In Seconds() -> (seconds since 1Jan1904=w260:timestamp)
            n257 = call-poly <vilib>:"Mean.vi"("X"=w267) -> ("mean"=w249:dbl)  [unwired: 1 out]
            n258 = call-poly <vilib>:"Mean.vi"("X"=w269) -> ("mean"=w250:dbl)  [unwired: 1 out]
            n259 = call-poly <vilib>:"Mean.vi"("X"=w271) -> ("mean"=w251:dbl)  [unwired: 1 out]
            n260 = call-poly <vilib>:"Mean.vi"("X"=w275) -> ("mean"=w252:dbl)  [unwired: 1 out]
            n261 = Get Date/Time String(seconds (now)=w260) -> (time string=→"time string":string)  [unwired: 2 in, 1 out]
            n262 = Build Array (concatenate)(w268, w250) -> (w263:dbl[])
            n263 = Build Array (concatenate)(w266, w249) -> (w261:dbl[])
            n264 = Build Array (concatenate)(w270, w251) -> (w264:dbl[])
            n265 = Build Array (concatenate)(w274, w252) -> (w273:dbl[])
            n266 = Build Array(w252, w251, w250, w249, w247) -> (w248:dbl[])
            "data array" <- w248
            n267 = Build Array (concatenate)(w276, w277) -> (w262:dbl[])
            n268 = Build Array (concatenate)(w281, w247) -> (w282:dbl[])
            n269 = call "Simple Temp Datalogger.vi"("data array"=w248, "datalog path (use dialog)"=path "C:/Temp/TEMPPOSOCT.DAT") -> ()  [unwired: 8 in]
            n270 = Bundle(w262, w261) -> (w253:cluster{dbl[], dbl[]})  [unwired: 1 in]
            n271 = Bundle(w262, w263) -> (w254:cluster{dbl[], dbl[]})  [unwired: 1 in]
            n272 = Bundle(w262, w264) -> (w255:cluster{dbl[], dbl[]})  [unwired: 1 in]
            n273 = Bundle(w262, w273) -> (w257:cluster{dbl[], dbl[]})  [unwired: 1 in]
            n274 = Bundle(w262, w282) -> (w256:cluster{dbl[], dbl[]})  [unwired: 1 in]
            n275 = Build Array(w253, w255, w254, w257, w256) -> (→"output cluster":cluster{dbl[], dbl[]}[])
          }
        }
        "Boolean" <- w172
        n276 = call "clearErrorMessageGUI.vi"("millisecond timer value"=w209, "Boolean"=w206, "error message"=w208, "reference"=w190) -> ("millisecond timer value 2"=w210:u32)
        n277 = call "StatusDataConnectionFGV.vi"("Command"=enum16{"get", "set", "init"}."get") -> ("Data Connection out"=→"image connection":bool)  [unwired: 10 in]
        n278 = call "StatusImageConnectionFGV.vi"("Command"=enum16{"get", "set", "init"}."get") -> ("Image Connection out"=→"data connection ok":bool)  [unwired: 10 in]
        "Image (IMAQ)" <- w164
        "Image (Guppy)" <- w160
        "Image (OAP)" <- w159
      }
      n279 = local read "connections (hidden)"() -> (w127:variant[])
      n280 = call "IMAQ Dispose"("Image"=w133) -> ()  [unwired: 5 in, 1 out]
      n281 = call "IMAQ Dispose"("Image"=w94) -> ()  [unwired: 5 in, 1 out]
      n282 = call "IMAQ Dispose"("Image"=w95) -> ()  [unwired: 5 in, 1 out]
      n283 = call "Close UDP AND TCP connections.vi"("error in"=w131, "appended array"=w127) -> ()  [unwired: 6 in]
    }
    frame #3 {
      n284 = flat-sequence {
        frame #0 {
          n285 = Wait (ms)(milliseconds to wait=u32 0) -> ()  [unwired: 1 out]
        }
        frame #1 {
          n286 = local write "stop"(FALSE ("stop")) -> ()
        }
        frame #2 {
          n287 = control-ref of="This VI"() -> (w466:refnum<vi>)
          n288 = case shown="True" FALSE {
            tunnel: w466 -> [w467 w470]
            tunnel: [w467 w468] -> w465
            frame False {
            }
            frame True {
              n289 = property class="VI" props=["Front Panel.Open"](reference=w470) -> (reference out=w469:refnum<vi>)  [unwired: 1 in, 2 out]
              n290 = invoke class="VI" method="FP.Close"(reference=w469) -> (reference out=w468:refnum<vi>)  [unwired: 2 in, 2 out]
            }
          }
          n291 = Close Reference(reference=w465) -> ()  [unwired: 1 in, 1 out]
        }
      }
      n292 = control-ref of="Main  Control"() -> (w460:refnum<vi>)
      n293 = property class="TabCtl (strict)"(reference=w460, "Tabs Visible?"=TRUE) -> ()  [unwired: 1 in, 2 out]
      n294 = property class="TabCtl (strict)"(reference=w460, "Tab Location"=enum32{"Top", "Bottom", "Left", "Right"}."Bottom") -> ()  [unwired: 1 in, 2 out]
    }
  }
